vi "Enable Output.vi"(8 "error in (no error)":errorcluster, 10 "Output Enable (F)":bool, 11 "PSG-MXG in":refnum<class "PSG-MXG.lvclass">) -> (0 "error out":errorcluster, 3 "PSG-MXG out":refnum<class "PSG-MXG.lvclass">)   [LabVIEW 2020, in "PSG-MXG.lvclass"]
uses:
  PSG-MXG.lvclass
  C:/Sandbox/RF Bench/Source Code/WiSpry Test Framework/Instruments/Instrument.lvclass
  C:/Sandbox/RF Bench/Source Code/WiSpry Test Framework/Instruments/Signal Generator/Signal Generator.lvclass
  Instrument.lvclass/Instrument.ctl
  Signal Generator.lvclass/Signal Generator.ctl
  Instrument.lvclass
  <instrlib>/Agilent PSG MXG Series/Agilent PSG MXG Series.lvlib
  Signal Generator.lvclass
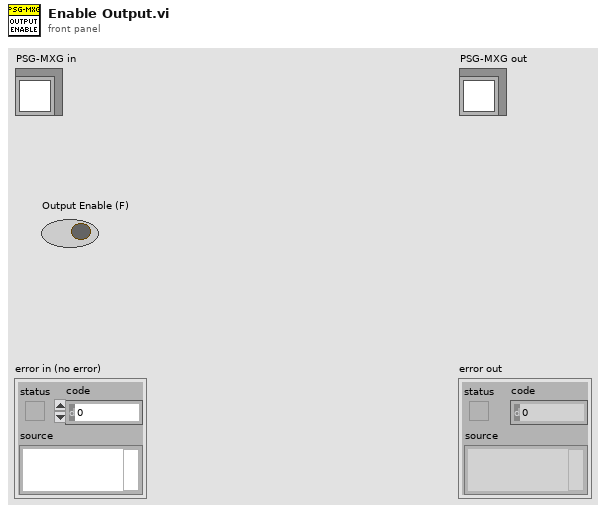
[diagram p1: front panel]
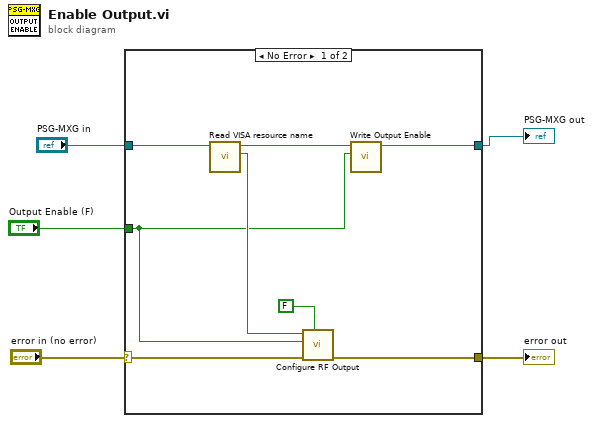
[diagram p0: block diagram]
diagram:
  n1 = case shown="No Error" "error in (no error)" {
    selector: "error in (no error)" -> [w12 w15]
    tunnel: "PSG-MXG in" -> [w13 w14]
    tunnel: [w11 w15] -> w4
    tunnel: [w6 w14] -> w3
    tunnel: "Output Enable (F)" -> [w8 _]
    frame No Error {
      n2 = call "Read VISA resource name.vi"("Instrument in"=w13) -> ("VISA resource name"=w10:refnum<visa-resource-name>, "Instrument out"=w7:refnum<class "PSG-MXG.lvclass">)  [unwired: 9 in]
      n3 = call <instrlib>:"Configure RF Output.vi"("Enable Modulation (T:Enable)"=FALSE, "error in (no error)"=w12, "Enable RF Output (F:Disable)"=w8, "VISA resource name"=w10) -> ("error out"=w11:errorcluster)  [unwired: 6 in, 1 out]
      n4 = call "Write Output Enable.vi"("Output Enable"=w8, "Signal Generator in"=w7) -> ("Signal Generator out"=w6:refnum<class "PSG-MXG.lvclass">)  [unwired: 9 in]
    }
    frame Error {
    }
  }
  "error out" <- w4
  "PSG-MXG out" <- w3
